vi "(Depricated) Launch Syringe Stepper.vi"(8 "error in (no error)":errorcluster, 11 "cRIO-CO2 in":refnum<class "cRIO-CO2.lvclass">) -> (0 "error out":errorcluster, 3 "cRIO-CO2 out":refnum<class "cRIO-CO2.lvclass">)   [LabVIEW 2015]
uses:
  cRIO-CO2 Messages/Log Message Msg/Log Message Msg.lvclass
  cRIO-CO2.lvclass
  Stepper/Stepper.lvclass
  <vilib>/ActorFramework/Actor/Actor.lvclass
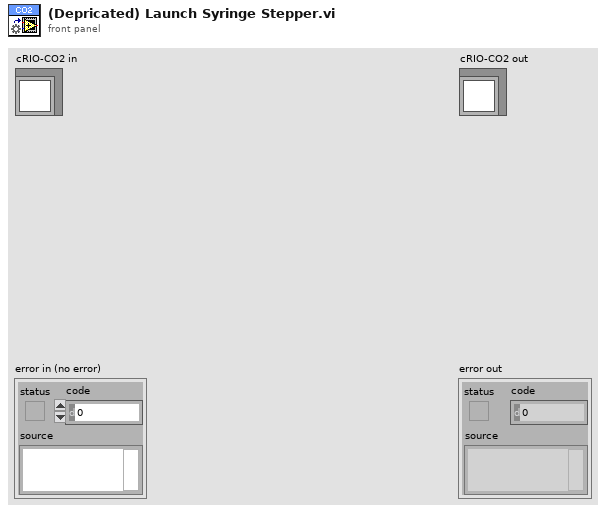
[diagram p1: front panel]
types:
  T1 = cluster{"Heater Duty Cycle SHV":refnum<k21>, "Thermocouple SHV":refnum<k21>, "Setpoint SHV":refnum<k21>, "Switch SHV":refnum<k21>}
  T2 = typedef "Dedicated Enqueuers.ctl" = cluster{"Freezers":cluster{"Syringe":refnum<class "Message Enqueuer.lvclass">, "Tank 1":refnum<class "Message Enqueuer.lvclass">, "Tank 2":refnum<class "Message Enqueuer.lvclass">, "Tank 3":refnum<class "Message Enqueuer.lvclass">, "Tank 4":refnum<class "Message Enqueuer.lvclass">}, "Heaters":cluster{"Syringe":refnum<class "Message Enqueuer.lvclass">, "Piston":refnum<class "Message Enqueuer.lvclass">}, "Blowers":cluster{"Tank 1":refnum<class "Message Enqueuer.lvclass">, "Tank 2":refnum<class "Message Enqueuer.lvclass">, "Tank 3":refnum<class "Message Enqueuer.lvclass">, "Tank 4":refnum<class "Message Enqueuer.lvclass">, "Syringe":refnum<class "Message Enqueuer.lvclass">}, "Sample Line":refnum<class "Message Enqueuer.lvclass">, "Storage Line":refnum<class "Message Enqueuer.lvclass">, "Transfer Line":refnum<class "Message Enqueuer.lvclass">, "Syringe Stepper":refnum<class "Message Enqueuer.lvclass">, "Syringe Line":refnum<class "Message Enqueuer.lvclass">, "Capillary Line":refnum<class "Message Enqueuer.lvclass">, "Preparation Line":refnum<class "Message Enqueuer.lvclass">, "Turbo":refnum<class "Message Enqueuer.lvclass">, "Vacuum":refnum<class "Message Enqueuer.lvclass">, "He Line":refnum<class "Message Enqueuer.lvclass">, "Cylinder":refnum<class "Message Enqueuer.lvclass">}
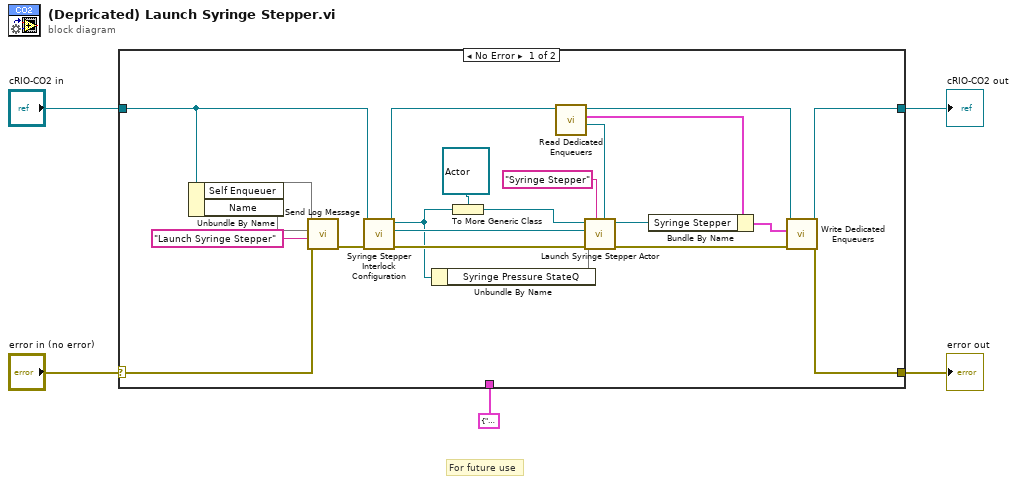
[diagram p0: block diagram]
diagram:
  # "For future use"
  n1 = case shown="No Error" "error in (no error)" {
    selector: "error in (no error)" -> [w24 w28]
    tunnel: [w14 w28] -> w4
    tunnel: [w18 w27] -> w2
    tunnel: "cRIO-CO2 in" -> [w21 w27]
    tunnel: T1 {"Heater Duty Cycle SHV"="ni.var.io://10.2.0.20/EtherCAT Master/Device/User-Defined Variables/Piston Heater Duty Cycle (‰)", "Thermocouple SHV"="ni.var.io://10.2.0.20/EtherCAT Master/Device/Mod2/Piston TC", "Setpoint SHV"="ni.var.psp://10.2.0.20/AMS Gas SHV/Heaters/Piston Heater Setpoint (C)", "Switch SHV"="ni.var.psp://10.2.0.20/AMS Gas SHV/Heaters/Piston Heater ON"} -> [_ _]
    frame No Error {
      n2 = Unbundle By Name(w21) -> ("Self Enqueuer"=w23, "Name"=w26)
      n3 = call "Send Log Message.vi"("error in (no error)"=w24, "String"="Launch Syringe Stepper", "Source Name"=w26, "Message Enqueuer"=w23) -> ("error out"=w22:errorcluster)  [unwired: 6 in, 1 out]
      n4 = call "Syringe Stepper Interlock Configuration.vi"("error in (no error)"=w22, "cRIO-CO2 in"=w21) -> ("error out"=w20:errorcluster, "Interlock Chain"=w19:refnum<class "Interlock Chain.lvclass">, "cRIO-CO2 out"=w7:refnum<class "cRIO-CO2.lvclass">)  [unwired: 7 in]
      n5 = Unbundle By Name(w7) -> ("Syringe Pressure StateQ"=w6)
      n6 = To More Generic Class(target class=refnum<class "Actor.lvclass"> refnum ("Caller Actor in"), reference=w7) -> (generic class reference=w13:refnum<class "Actor.lvclass">)
      n7 = call "Read Dedicated Enqueuers.vi"("cRIO-CO2 in"=w7) -> ("Qs.DedicatedEnQrs"=w9:refnum<queue>, "Dedicated Enqueuers"=w17:T2, "cRIO-CO2 out"=w8:refnum<class "cRIO-CO2.lvclass">)  [unwired: 7 in, 1 out]
      n8 = call "Launch Syringe Stepper Actor.vi"("DedicatedEnQrs"=w9, "Name"="Syringe Stepper", "error in (no error)"=w20, "Syringe Pressure StateQ"=w6, "Interlock Chain"=w19, "Caller Actor in"=w13) -> ("error out"=w10:errorcluster, "Caller-To-Actor Enqueuer"=w15:refnum<class "Message Enqueuer.lvclass">)  [unwired: 4 in]
      n9 = Bundle By Name(cluster=w17, "Syringe Stepper"=w15) -> (w16:T2)
      n10 = call "Write Dedicated Enqueuers.vi"("error in (no error)"=w10, "Dedicated Enqueuers"=w16, "cRIO-CO2 in"=w8) -> ("error out"=w14:errorcluster, "cRIO-CO2 out"=w18:refnum<class "cRIO-CO2.lvclass">)  [unwired: 7 in]
    }
    frame Error {
    }
  }
  "error out" <- w4
  "cRIO-CO2 out" <- w2
